vi "Constructor.vi"(10 "Beverage":refnum<class "Beverage.lvclass">, 11 "Whip in":refnum<class "Whip.lvclass">) -> (3 "Whip out":refnum<class "Whip.lvclass">)   [LabVIEW 2011, in "Whip.lvclass"]
uses:
  Whip.lvclass
  Beverage/Beverage.lvclass
  Whip.lvclass/Whip.ctl
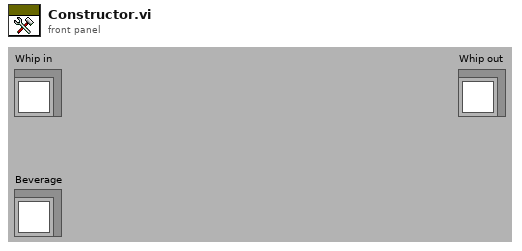
[diagram p1: front panel]
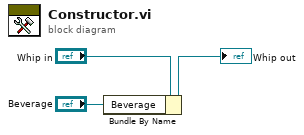
[diagram p0: block diagram]
diagram:
  n1 = Bundle By Name(cluster="Whip in", "Beverage"="Beverage") -> (→"Whip out":refnum<class "Whip.lvclass">)
